vi "Sub UI Update basic point.vi"(8 "error in (no error)":errorcluster, 11 "LF2R IDE in":refnum<class "LF2R IDE.lvclass">) -> (0 "error out":errorcluster, 3 "LF2R IDE out":refnum<class "LF2R IDE.lvclass">)   [LabVIEW 2018, in "LF2R IDE.lvlib" / "LF2R IDE.lvclass"]
uses:
  LF2R IDE.lvclass
  LF2R IDE.lvclass/LF2R IDE.ctl
  Image/Image Process.lvclass
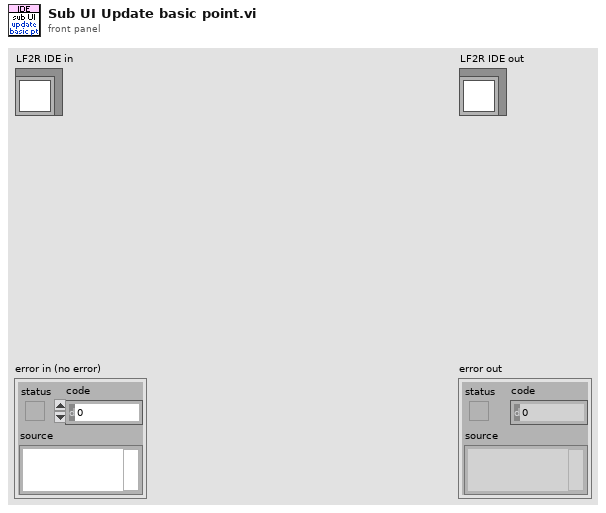
[diagram p1: front panel]
types:
  T1 = typedef "IMAQ Image.ctl" = refnum<image>
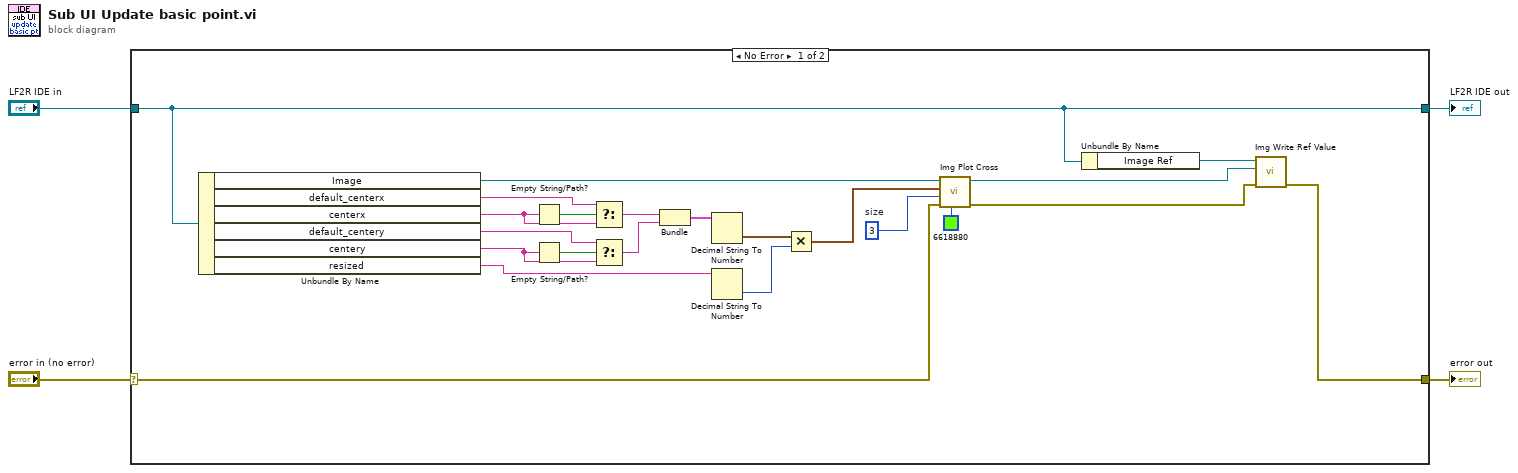
[diagram p0: block diagram]
diagram:
  n1 = case shown="No Error" "error in (no error)" {
    selector: "error in (no error)" -> [w9 w28]
    tunnel: [w24 w28] -> w3
    tunnel: [w26 w27] -> w1
    tunnel: "LF2R IDE in" -> [w26 w27]
    frame No Error {
      w8 = 3  # size
      n2 = Unbundle By Name(w26) -> ("Image"=w11:T1, "default_centerx"=w19:string, "centerx"=w18:string, "default_centery"=w16:string, "centery"=w15:string, "resized"=w23:string)
      n3 = Empty String/Path?(string/path=w18) -> (empty?=w20:bool)
      n4 = Empty String/Path?(string/path=w15) -> (empty?=w17:bool)
      n5 = Select(t=w19, s=w20, f=w18) -> (s? t:f=w14:string)
      n6 = Select(t=w16, s=w17, f=w15) -> (s? t:f=w13:string)
      n7 = Bundle("centerx"=w14, "centery"=w13) -> (w12:cluster{"centerx":string, "centery":string})  [unwired: 1 in]
      n8 = Decimal String To Number(string=w12) -> (number=w22:cluster{"centerx":i32, "centery":i32})  [unwired: 2 in, 1 out]
      n9 = Decimal String To Number(string=w23) -> (number=w21:i32)  [unwired: 2 in, 1 out]
      n10 = Multiply(x=w22, y=w21) -> (x*y=w10:cluster{"centerx":i32, "centery":i32})
      n11 = call "Img Plot Cross.vi"("Color"=u32 6618880, "error in (no error)"=w9, "size"=w8, "position"=w10, "Image In"=w11) -> ("error out"=w6:errorcluster, "Image Out"=w5:T1)  [unwired: 5 in]
      n12 = Unbundle By Name(w26) -> ("Image Ref"=w25:refnum<vi>)
      n13 = call "Img Write Ref Value.vi"("error in (no error)"=w6, "Image"=w5, "Image Ref"=w25) -> ("error out"=w24:errorcluster)  [unwired: 8 in]
    }
    frame Error {
    }
  }
  "error out" <- w3
  "LF2R IDE out" <- w1
